vi "Get RIO Resource.vi"(8 "error in":errorcluster, 11 "FPGA addon refnum in":T1=18446744073709551615 format="%.0x") -> (0 "error out":errorcluster, 2 "RIO resource":string, 3 "FPGA addon refnum out":T1=18446744073709551615 format="%.0x")   [LabVIEW 2019, in "Scripting API.lvlib"]
doc: "Returns the hardware RIO resource configured for the target FPGA addon custom device."
uses:
  Scripting API.lvlib
  <vilib>/NI VeriStand/Custom Device API/Custom Device Item Ref.ctl
  Addon/Addon Shared/Types/FG Action.ctl
  Addon/Addon Shared/SubVIs/Constants.vi
  <vilib>/NI VeriStand/Custom Device API/NI VeriStand - Get Item Property.vi
  <vilib>/NI VeriStand/Custom Device API/Get Item Property (Path).vi
  <vilib>/NI VeriStand/Custom Device API/Get Item Property (String).vi
  <vilib>/NI VeriStand/Custom Device API/Get Item Property (Boolean).vi
  <vilib>/NI VeriStand/Custom Device API/NI VeriStand - Set Item Property.vi
  <vilib>/NI VeriStand/Custom Device API/Set Item Property (Path).vi
  <vilib>/NI VeriStand/Custom Device API/Set Item Property (String).vi
  <vilib>/NI VeriStand/Custom Device API/Set Item Property (Boolean).vi
  Addon/Addon Shared/FPGA Addon Shared.lvlib
  <vilib>/NI VeriStand/Custom Device API/Custom Device API.lvlib
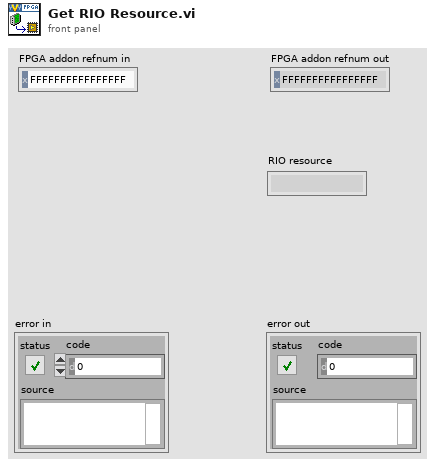
[diagram p1: front panel]
types:
  T1 = typedef "Custom Device API.lvlib/Custom Device Item Ref.ctl" = u64
  T2 = typedef "FPGA Addon Shared.lvlib/FG Action.ctl" = enum8{"GET", "SET"}
  T3 = typedef "FPGA Addon Shared.lvlib/FPGA Settings.ctl" = cluster{"Bitfile path":path, "RIO Device Address":string, "Group":bool}
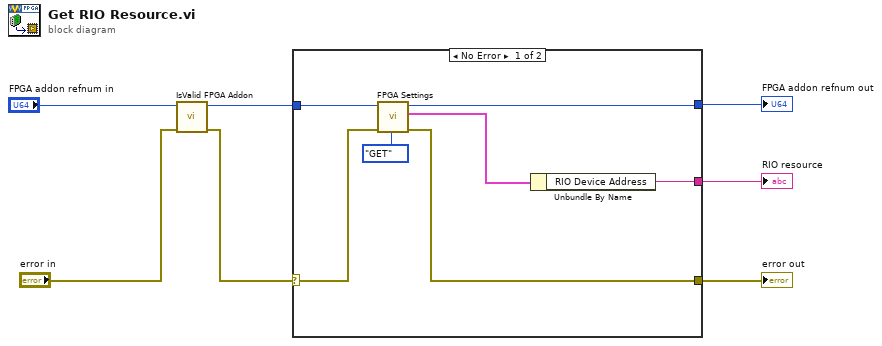
[diagram p0: block diagram]
diagram:
  n1 = call "IsValid FPGA Addon.vi"("error in"="error in", "FPGA Addon refnum in"="FPGA addon refnum in") -> ("error out"=w6:errorcluster, "FPGA Addon refnum out"=w7:T1)  [unwired: 8 in]
  n2 = case shown="No Error" w6 {
    selector: w6 -> [w12 w15]
    tunnel: w7 -> [w14 w16]
    tunnel: [w8 w15] -> w3
    tunnel: [w10 w16] -> w4
    tunnel: [w9 _] -> w1
    frame No Error {
      n3 = call "FPGA Settings.vi"("Action"=FG_Action."GET", "error in (no error)"=w12, "Item Ref"=w14) -> ("error out"=w8:errorcluster, "FPGA Settings"=w11:T3, "Item Ref out"=w10:T1)  [unwired: 6 in]
      n4 = Unbundle By Name(w11) -> ("RIO Device Address"=w9:string)
    }
    frame Error {
    }
  }
  "error out" <- w3
  "FPGA addon refnum out" <- w4
  "RIO resource" <- w1
